vi "Check Bookmarks.vi"(5 "Exclude Bookmarks":string[](array[string]), 7 "Include Bookmarks":string[](array[string]), 8 "error in (no error)":errorcluster, 10 "App Ref":refnum<vi>, 11 "VI Path":path) -> (0 "error out":errorcluster, 2 "Check If Unit Test?":bool, 3 "VI Path dup":path)   [LabVIEW 2023]
doc: "Checks VI bookmarks against a list of Include and Exclude bookmarks.\n\nIf there is an Include list, then only run the Unit Test if a VI contains a bookmark in the list. \nIf there is an Exclude list, then do not run the Unit Test if the VI contains a bookmark in the list. \n\nIf both list, then a VI must contain a bookmark from the Include list while also not containing a bookmark from the Exclude list."
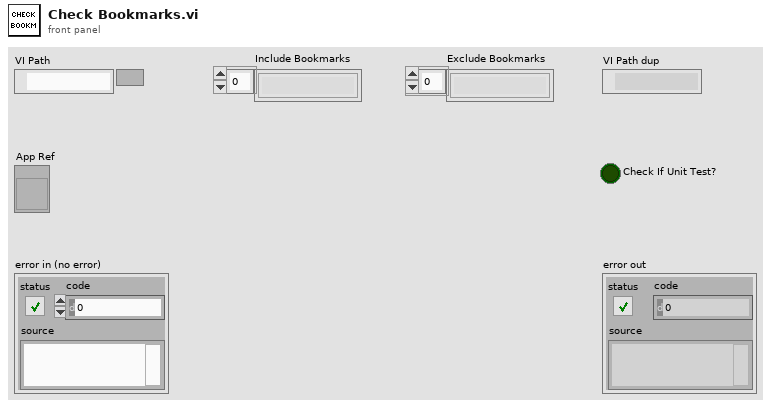
[diagram p1: front panel]
types:
  T1 = typedef "LVBookmarkInfoTypeDef.ctl" = cluster{"Bookmark Reference":u32, "Bookmark Tag":string, "Label Text":string}[]
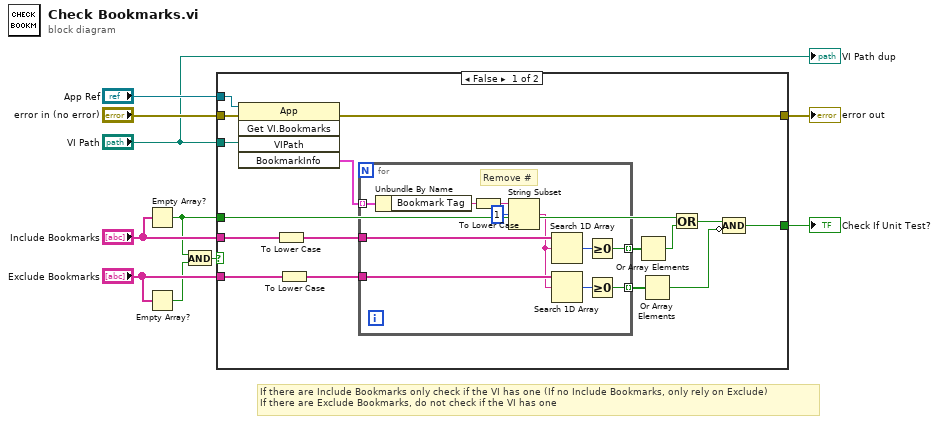
[diagram p0: block diagram]
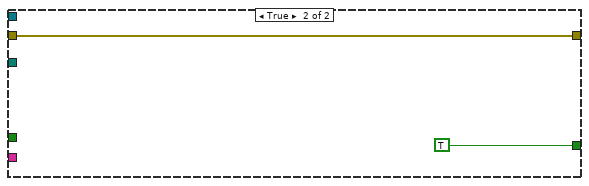
[diagram p2: hidden frame]
diagram:
  # "If there are Include Bookmarks only check if the VI has one (If no Include Bookmarks, only rely on Exclude)\nIf there are Exclude Bookmarks, do not check if the VI has one"
  n1 = Empty Array?(array="Include Bookmarks") -> (empty?=w3:bool)
  n2 = Empty Array?(array="Exclude Bookmarks") -> (empty?=w6:bool)
  n3 = And(x=w3, y=w6) -> (x .and. y?=w5:bool)
  n4 = case shown="False" w5 {
    tunnel: [w15 w39] -> w10
    tunnel: "error in (no error)" -> [w14 w39]
    tunnel: "Include Bookmarks" -> [w24 _]
    tunnel: "Exclude Bookmarks" -> [w23 _]
    tunnel: [w21 TRUE] -> w4
    tunnel: w3 -> [w20 _]
    tunnel: "App Ref" -> [w12 _]
    tunnel: "VI Path" -> [w11 _]
    frame False {
      n5 = invoke class="App" method="Get VI.Bookmarks"(reference=w12, error in=w14, "VIPath"=w11) -> (error out=w15:errorcluster, "BookmarkInfo"=w13:T1)  [unwired: 2 in, 3 out]
      n6 = To Lower Case(string=w24) -> (all lower case string=w17:string[])
      n7 = To Lower Case(string=w23) -> (all lower case string=w16:string[])
      n8 = for {
        tunnel: w13 -> [w37] mode=indexing
        tunnel: w17 -> [w36]
        tunnel: w16 -> [w35]
        tunnel: [w32] -> w25 mode=indexing
        tunnel: [w31] -> w26 mode=indexing
        # "Remove #"
        n9 = Unbundle By Name(w37) -> ("Bookmark Tag"=w30:string)
        n10 = To Lower Case(string=w30) -> (all lower case string=w27:string)
        n11 = String Subset(string=w27, offset (0)=1) -> (substring=w29:string)  [unwired: 1 in]
        n12 = Search 1D Array(1D array=w36, element=w29) -> (index of element=w34:i32)  [unwired: 1 in]
        n13 = Search 1D Array(1D array=w35, element=w29) -> (index of element=w33:i32)  [unwired: 1 in]
        n14 = Greater Or Equal To 0?(x=w34) -> (x >= 0?=w31:bool)
        n15 = Greater Or Equal To 0?(x=w33) -> (x >= 0?=w32:bool)
      }
      n16 = Or Array Elements(Boolean array=w26) -> (logical OR=w19:bool)
      n17 = Or Array Elements(Boolean array=w25) -> (logical OR=w22:bool)
      n18 = Or(x=w20, y=w19) -> (x .or. y?=w18:bool)
      n19 = Compound Arithmetic op=AND(w18, invert w22) -> (w21:bool)
    }
    frame True {
    }
  }
  "error out" <- w10
  "Check If Unit Test?" <- w4
  "VI Path dup" <- "VI Path"
